vi "ABCtoAlphaBeta_2PhasePowerInvariant_src.vi"(0 "A":sgl, 5 "B":sgl) -> (4 "alpha":sgl, 6 "beta":sgl)   [LabVIEW 2017]
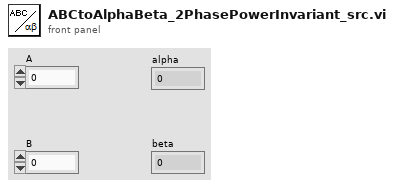
[diagram p1: front panel]
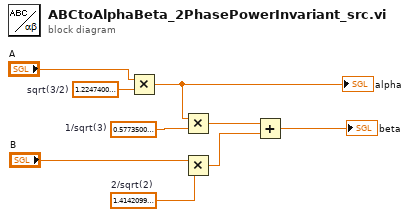
[diagram p0: block diagram]
diagram:
  w4 = sgl 1.22474  # sqrt(3/2)
  w5 = sgl 1.41421  # 2/sqrt(2)
  w6 = sgl 0.57735  # 1/sqrt(3)
  n1 = Multiply(x="A", y=w4) -> (x*y=w2:sgl)
  "alpha" <- w2
  n2 = Multiply(x=w2, y=w6) -> (x*y=w9:sgl)
  n3 = Multiply(x="B", y=w5) -> (x*y=w8:sgl)
  n4 = Add(x=w9, y=w8) -> (x+y=→"beta":sgl)
